vi "GeoData.vi"() -> ()   [LabVIEW 2017] (continued)
H1\n49649\t26055\tKingsley\tMI\tGrand Traverse County\tH1\n49684\t26055\tTraverse city\tMI\tGrand Traverse County\tH1\n49696\t26055\tTraverse city\tMI\tGrand Traverse County\tH1\n49666\t26055\tMayfield\tMI\tGrand Traverse County\tH1\n49683\t26055\tThompsonville\tMI\tGrand Traverse County\tH1\n48811\t26057\tCarson city\tMI\tGratiot County\tH1\n48862\t26057\tNorth star\tMI\tGratiot County\tH1\n48818\t26057\tCrystal\tMI\tGratiot County\tH1\n48830\t26057\tElm hall\tMI\tGratiot County\tH1\n48806\t26057\tAshley\tMI\tGratiot County\tH1\n48877\t26057\tRiverdale\tMI\tGratiot County\tH1\n48847\t26057\tIthaca\tMI\tGratiot County\tH1\n48874\t26057\tPompeii\tMI\tGratiot County\tH1\n48883\t26057\tShepherd\tMI\tGratiot County\tH1\n48891\t26057\tVestaburg\tMI\tGratiot County\tH1\n48879\t26057\tSaint johns\tMI\tGratiot County\tH1\n48889\t26057\tSumner\tMI\tGratiot County\tH1\n48637\t26057\tMerrill\tMI\tGratiot County\tH1\n48845\t26057\tHubbardston\tMI\tGratiot County\tH1\n48880\t26057\tSaint louis\tMI\tGratiot County\tH1\n48835\t26057\tFowler\tMI\tGratiot County\tH1\n48615\t26057\tBreckenridge\tMI\tGratiot County\tH1\n48832\t26057\tElwell\tMI\tGratiot County\tH1\n48801\t26057\tAlma\tMI\tGratiot County\tH1\n48662\t26057\tWheeler\tMI\tGratiot County\tH1\n48856\t26057\tMiddleton\tMI\tGratiot County\tH1\n48871\t26057\tPerrinton\tMI\tGratiot County\tH1\n48807\t26057\tBannister\tMI\tGratiot County\tH1\n48614\t26057\tBrant\tMI\tGratiot County\tH1\n48831\t26057\tElsie\tMI\tGratiot County\tH1\n49262\t26059\tNorth adams\tMI\tHillsdale County\tH1\n49255\t26059\tMontgomery\tMI\tHillsdale County\tH1\n49082\t26059\tQuincy\tMI\tHillsdale County\tH1\n49246\t26059\tHorton\tMI\tHillsdale County\tH1\n49220\t26059\tAddison\tMI\tHillsdale County\tH1\n49250\t26059\tJonesville\tMI\tHillsdale County\tH1\n49274\t26059\tReading\tMI\tHillsdale County\tH1\n49245\t26059\tHomer\tMI\tHillsdale County\tH1\n49282\t26059\tSomerset center\tMI\tHillsdale County\tH1\n49252\t26059\tLitchfield\tMI\tHillsdale County\tH1\n49233\t26059\tCement city\tMI\tHillsdale County\tH1\n49258\t26059\tMosherville\tMI\tHillsdale County\tH1\n49242\t26059\tHillsdale\tMI\tHillsdale County\tH1\n49266\t26059\tOsseo\tMI\tHillsdale County\tH1\n49249\t26059\tJerome\tMI\tHillsdale County\tH1\n49271\t26059\tPittsford\tMI\tHillsdale County\tH1\n49288\t26059\tWaldron\tMI\tHillsdale County\tH1\n49239\t26059\tFrontier\tMI\tHillsdale County\tH1\n49232\t26059\tCamden\tMI\tHillsdale County\tH1\n49227\t26059\tAllen\tMI\tHillsdale County\tH1\n49241\t26059\tHanover\tMI\tHillsdale County\tH1\n49247\t26059\tHudson\tMI\tHillsdale County\tH1\n49257\t26059\tMoscow\tMI\tHillsdale County\tH1\n49281\t26059\tSomerset\tMI\tHillsdale County\tH1\n49931\t26061\tHoughton\tMI\tHoughton County\tH1\n49901\t26061\tAhmeek\tMI\tHoughton County\tH1\n49916\t26061\tChassell\tMI\tHoughton County\tH1\n49967\t26061\tTrout creek\tMI\tHoughton County\tH1\n49921\t26061\tDodgeville\tMI\tHoughton County\tH1\n49930\t26061\tHancock\tMI\tHoughton County\tH1\n49905\t26061\tAtlantic mine\tMI\tHoughton County\tH1\n49963\t26061\tSouth range\tMI\tHoughton County\tH1\n49952\t26061\tNisula\tMI\tHoughton County\tH1\n49961\t26061\tSidnaw\tMI\tHoughton County\tH1\n49958\t26061\tPelkie\tMI\tHoughton County\tH1\n49917\t26061\tCopper city\tMI\tHoughton County\tH1\n49934\t26061\tHubbell\tMI\tHoughton County\tH1\n49945\t26061\tLake linden\tMI\tHoughton County\tH1\n49913\t26061\tCalumet\tMI\tHoughton County\tH1\n49805\t26061\tAllouez\tMI\tHoughton County\tH1\n49922\t26061\tDollar bay\tMI\tHoughton County\tH1\n49965\t26061\tToivola\tMI\tHoughton County\tH1\n49955\t26061\tPainesdale\tMI\tHoughton County\tH1\n48413\t26063\tBad axe\tMI\tHuron County\tH1\n48456\t26063\tMinden city\tMI\tHuron County\tH1\n48726\t26063\tCass city\tMI\tHuron County\tH1\n48720\t26063\tBay port\tMI\tHuron County\tH1\n48755\t26063\tPigeon\tMI\tHuron County\tH1\n48725\t26063\tCaseville\tMI\tHuron County\tH1\n48731\t26063\tElkton\tMI\tHuron County\tH1\n48735\t26063\tGagetown\tMI\tHuron County\tH1\n48467\t26063\tPort austin\tMI\tHuron County\tH1\n48470\t26063\tRuth\tMI\tHuron County\tH1\n48445\t26063\tKinde\tMI\tHuron County\tH1\n48759\t26063\tSebewaing\tMI\tHuron County\tH1\n48754\t26063\tOwendale\tMI\tHuron County\tH1\n48468\t26063\tPort hope\tMI\tHuron County\tH1\n48441\t26063\tHarbor beach\tMI\tHuron County\tH1\n48475\t26063\tUbly\tMI\tHuron County\tH1\n48432\t26063\tFilion\tMI\tHuron County\tH1\n48767\t26063\tUnionville\tMI\tHuron County\tH1\n49285\t26065\tStockbridge\tMI\tIngham County\tH1\n48826\t26065\tEast lansing\tMI\tIngham County\tH1\n48933\t26065\tLansing\tMI\tIngham County\tH1\n48805\t26065\tOkemos\tMI\tIngham County\tH1\n48864\t26065\tOkemos\tMI\tIngham County\tH1\n48840\t26065\tHaslett\tMI\tIngham County\tH1\n48824\t26065\tEast lansing\tMI\tIngham County\tH1\n48854\t26065\tMason\tMI\tIngham County\tH1\n48821\t26065\tDimondale\tMI\tIngham County\tH1\n48924\t26065\tLansing\tMI\tIngham County\tH1\n48911\t26065\tLansing\tMI\tIngham County\tH1\n48917\t26065\tLansing\tMI\tIngham County\tH1\n48825\t26065\tEast lansing\tMI\tIngham County\tH1\n48892\t26065\tWebberville\tMI\tIngham County\tH1\n48842\t26065\tHolt\tMI\tIngham County\tH1\n48819\t26065\tDansville\tMI\tIngham County\tH1\n48906\t26065\tLansing\tMI\tIngham County\tH1\n48909\t26065\tLansing\tMI\tIngham County\tH1\n48915\t26065\tLansing\tMI\tIngham County\tH1\n49264\t26065\tOnondaga\tMI\tIngham County\tH1\n48823\t26065\tEast lansing\tMI\tIngham County\tH1\n48910\t26065\tLansing\tMI\tIngham County\tH1\n48872\t26065\tPerry\tMI\tIngham County\tH1\n48901\t26065\tLansing\tMI\tIngham County\tH1\n48956\t26065\tLansing\tMI\tIngham County\tH1\n49251\t26065\tLeslie\tMI\tIngham County\tH1\n48827\t26065\tEaton rapids\tMI\tIngham County\tH1\n48912\t26065\tLansing\tMI\tIngham County\tH1\n48895\t26065\tWilliamston\tMI\tIngham County\tH1\n48849\t26067\tLake odessa\tMI\tIonia County\tH1\n48860\t26067\tMuir\tMI\tIonia County\tH1\n49331\t26067\tLowell\tMI\tIonia County\tH1\n49325\t26067\tFreeport\tMI\tIonia County\tH1\n48846\t26067\tIonia\tMI\tIonia County\tH1\n48875\t26067\tPortland\tMI\tIonia County\tH1\n48881\t26067\tSaranac\tMI\tIonia County\tH1\n48809\t26067\tBelding\tMI\tIonia County\tH1\n48838\t26067\tGreenville\tMI\tIonia County\tH1\n48890\t26067\tSunfield\tMI\tIonia County\tH1\n48834\t26067\tFenwick\tMI\tIonia County\tH1\n48815\t26067\tClarksville\tMI\tIonia County\tH1\n48865\t26067\tOrleans\tMI\tIonia County\tH1\n48873\t26067\tPewamo\tMI\tIonia County\tH1\n48870\t26067\tPalo\tMI\tIonia County\tH1\n48845\t26067\tHubbardston\tMI\tIonia County\tH1\n48894\t26067\tWestphalia\tMI\tIonia County\tH1\n48837\t26067\tGrand ledge\tMI\tIonia County\tH1\n48851\t26067\tLyons\tMI\tIonia County\tH1\n48861\t26067\tMulliken\tMI\tIonia County\tH1\n49302\t26067\tAlto\tMI\tIonia County\tH1\n48750\t26069\tOscoda\tMI\tIosco County\tH1\n48748\t26069\tNational city\tMI\tIosco County\tH1\n48770\t26069\tWhittemore\tMI\tIosco County\tH1\n48739\t26069\tHale\tMI\tIosco County\tH1\n48766\t26069\tTwining\tMI\tIosco County\tH1\n48761\t26069\tSouth branch\tMI\tIosco County\tH1\n48745\t26069\tMikado\tMI\tIosco County\tH1\n48738\t26069\tGreenbush\tMI\tIosco County\tH1\n48737\t26069\tGlennie\tMI\tIosco County\tH1\n48765\t26069\tTurner\tMI\tIosco County\tH1\n48730\t26069\tEast tawas\tMI\tIosco County\tH1\n48763\t26069\tTawas city\tMI\tIosco County\tH1\n48743\t26069\tLong lake\tMI\tIosco County\tH1\n49967\t26071\tTrout creek\tMI\tIron County\tH1\n49915\t26071\tCaspian\tMI\tIron County\tH1\n49927\t26071\tGaastra\tMI\tIron County\tH1\n49902\t26071\tAlpha\tMI\tIron County\tH1\n49920\t26071\tCrystal falls\tMI\tIron County\tH1\n49903\t26071\tAmasa\tMI\tIron County\tH1\n49879\t26071\tRepublic\tMI\tIron County\tH1\n49935\t26071\tIron river\tMI\tIron County\tH1\n49964\t26071\tStambaugh\tMI\tIron County\tH1\n48632\t26073\tLake\tMI\tIsabella County\tH1\n48804\t26073\tMount pleasant\tMI\tIsabella County\tH1\n49310\t26073\tBlanchard\tMI\tIsabella County\tH1\n49340\t26073\tRemus\tMI\tIsabella County\tH1\n49305\t26073\tBarryton\tMI\tIsabella County\tH1\n48618\t26073\tColeman\tMI\tIsabella County\tH1\n48877\t26073\tRiverdale\tMI\tIsabella County\tH1\n48893\t26073\tWeidman\tMI\tIsabella County\tH1\n48878\t26073\tRosebush\tMI\tIsabella County\tH1\n48622\t26073\tFarwell\tMI\tIsabella County\tH1\n48883\t26073\tShepherd\tMI\tIsabella County\tH1\n48891\t26073\tVestaburg\tMI\tIsabella County\tH1\n48858\t26073\tMount pleasant\tMI\tIsabella County\tH1\n48880\t26073\tSaint louis\tMI\tIsabella County\tH1\n48896\t26073\tWinn\tMI\tIsabella County\tH1\n48617\t26073\tClare\tMI\tIsabella County\tH1\n48801\t26073\tAlma\tMI\tIsabella County\tH1\n48829\t26073\tEdmore\tMI\tIsabella County\tH1\n48859\t26073\tMount pleasant\tMI\tIsabella County\tH1\n49224\t26075\tAlbion\tMI\tJackson County\tH1\n49202\t26075\tJackson\tMI\tJackson County\tH1\n49285\t26075\tStockbridge\tMI\tJackson County\tH1\n49272\t26075\tPleasant lake\tMI\tJackson County\tH1\n49203\t26075\tJackson\tMI\tJackson County\tH1\n49246\t26075\tHorton\tMI\tJackson County\tH1\n49204\t26075\tJackson\tMI\tJackson County\tH1\n49250\t26075\tJonesville\tMI\tJackson County\tH1\n49245\t26075\tHomer\tMI\tJackson County\tH1\n49201\t26075\tJackson\tMI\tJackson County\tH1\n49269\t26075\tParma\tMI\tJackson County\tH1\n49277\t26075\tRives junction\tMI\tJackson County\tH1\n49252\t26075\tLitchfield\tMI\tJackson County\tH1\n49284\t26075\tSpringport\tMI\tJackson County\tH1\n49259\t26075\tMunith\tMI\tJackson County\tH1\n49233\t26075\tCement city\tMI\tJackson County\tH1\n48158\t26075\tManchester\tMI\tJackson County\tH1\n49237\t26075\tConcord\tMI\tJackson County\tH1\n49254\t26075\tMichigan center\tMI\tJackson County\tH1\n49263\t26075\tNorvell\tMI\tJackson County\tH1\n48118\t26075\tChelsea\tMI\tJackson County\tH1\n49234\t26075\tClarklake\tMI\tJackson County\tH1\n49249\t26075\tJerome\tMI\tJackson County\tH1\n49261\t26075\tNapoleon\tMI\tJackson County\tH1\n49264\t26075\tOnondaga\tMI\tJackson County\tH1\n49241\t26075\tHanover\tMI\tJackson County\tH1\n49230\t26075\tBrooklyn\tMI\tJackson County\tH1\n49240\t26075\tGrass lake\tMI\tJackson County\tH1\n49251\t26075\tLeslie\tMI\tJackson County\tH1\n49283\t26075\tSpring arbor\tMI\tJackson County\tH1\n48827\t26075\tEaton rapids\tMI\tJackson County\tH1\n49004\t26077\tKalamazoo\tMI\tKalamazoo County\tH1\n49080\t26077\tPlainwell\tMI\tKalamazoo County\tH1\n49074\t26077\tNazareth\tMI\tKalamazoo County\tH1\n49009\t26077\tKalamazoo\tMI\tKalamazoo County\tH1\n49007\t26077\tKalamazoo\tMI\tKalamazoo County\tH1\n49083\t26077\tRichland\tMI\tKalamazoo County\tH1\n49087\t26077\tSchoolcraft\tMI\tKalamazoo County\tH1\n49003\t26077\tKalamazoo\tMI\tKalamazoo County\tH1\n49060\t26077\tHickory corners\tMI\tKalamazoo County\tH1\n49011\t26077\tAthens\tMI\tKalamazoo County\tH1\n49008\t26077\tKalamazoo\tMI\tKalamazoo County\tH1\n49072\t26077\tMendon\tMI\tKalamazoo County\tH1\n49005\t26077\tKalamazoo\tMI\tKalamazoo County\tH1\n49034\t26077\tClimax\tMI\tKalamazoo County\tH1\n49006\t26077\tKalamazoo\tMI\tKalamazoo County\tH1\n49015\t26077\tBattle creek\tMI\tKalamazoo County\tH1\n49001\t26077\tKalamazoo\tMI\tKalamazoo County\tH1\n49097\t26077\tVicksburg\tMI\tKalamazoo County\tH1\n49065\t26077\tLawton\tMI\tKalamazoo County\tH1\n49078\t26077\tOtsego\tMI\tKalamazoo County\tH1\n49052\t26077\tFulton\tMI\tKalamazoo County\tH1\n49053\t26077\tGalesburg\tMI\tKalamazoo County\tH1\n49081\t26077\tPortage\tMI\tKalamazoo County\tH1\n49041\t26077\tComstock\tMI\tKalamazoo County\tH1\n49017\t26077\tBattle creek\tMI\tKalamazoo County\tH1\n49037\t26077\tBattle creek\tMI\tKalamazoo County\tH1\n49012\t26077\tAugusta\tMI\tKalamazoo County\tH1\n49019\t26077\tKalamazoo\tMI\tKalamazoo County\tH1\n49024\t26077\tPortage\tMI\tKalamazoo County\tH1\n49002\t26077\tPortage\tMI\tKalamazoo County\tH1\n49048\t26077\tKalamazoo\tMI\tKalamazoo County\tH1\n49071\t26077\tMattawan\tMI\tKalamazoo County\tH1\n49088\t26077\tScotts\tMI\tKalamazoo County\tH1\n49077\t26077\tOshtemo\tMI\tKalamazoo County\tH1\n49690\t26079\tWilliamsburg\tMI\tKalkaska County\tH1\n49680\t26079\tSouth boardman\tMI\tKalkaska County\tH1\n49612\t26079\tAlden\tMI\tKalkaska County\tH1\n49633\t26079\tFife lake\tMI\tKalkaska County\tH1\n49659\t26079\tMancelona\tMI\tKalkaska County\tH1\n49738\t26079\tGrayling\tMI\tKalkaska County\tH1\n49646\t26079\tKalkaska\tMI\tKalkaska County\tH1\n49676\t26079\tRapid city\tMI\tKalkaska County\tH1\n49323\t26081\tDorr\tMI\tKent County\tH1\n49331\t26081\tLowell\tMI\tKent County\tH1\n49325\t26081\tFreeport\tMI\tKent County\tH1\n49418\t26081\tGrandville\tMI\tKent County\tH1\n49515\t26081\tGrand rapids\tMI\tKent County\tH1\n49514\t26081\tGrand rapids\tMI\tKent County\tH1\n49351\t26081\tRockford\tMI\tKent County\tH1\n49519\t26081\tWyoming\tMI\tKent County\tH1\n49507\t26081\tGrand rapids\tMI\tKent County\tH1\n49348\t26081\tWayland\tMI\tKent County\tH1\n49504\t26081\tGrand rapids\tMI\tKent County\tH1\n49518\t26081\tGrand rapids\tMI\tKent County\tH1\n49588\t26081\tGrand rapids\tMI\tKent County\tH1\n49315\t26081\tByron center\tMI\tKent County\tH1\n49330\t26081\tKent city\tMI\tKent County\tH1\n49316\t26081\tCaledonia\tMI\tKent County\tH1\n49534\t26081\tGrand rapids\tMI\tKent County\tH1\n49509\t26081\tWyoming\tMI\tKent County\tH1\n49508\t26081\tGrand rapids\tMI\tKent County\tH1\n49546\t26081\tGrand rapids\tMI\tKent County\tH1\n49544\t26081\tGrand rapids\tMI\tKent County\tH1\n49326\t26081\tGowen\tMI\tKent County\tH1\n48809\t26081\tBelding\tMI\tKent County\tH1\n48838\t26081\tGreenville\tMI\tKent County\tH1\n49319\t26081\tCedar springs\tMI\tKent County\tH1\n49506\t26081\tGrand rapids\tMI\tKent County\tH1\n49525\t26081\tGrand rapids\tMI\tKent County\tH1\n49345\t26081\tSparta\tMI\tKent County\tH1\n48815\t26081\tClarksville\tMI\tKent County\tH1\n49347\t26081\tTrufant\tMI\tKent County\tH1\n49321\t26081\tComstock park\tMI\tKent County\tH1\n49327\t26081\tGrant\tMI\tKent County\tH1\n49301\t26081\tAda\tMI\tKent County\tH1\n49512\t26081\tGrand rapids\tMI\tKent County\tH1\n49516\t26081\tGrand rapids\tMI\tKent County\tH1\n49343\t26081\tSand lake\tMI\tKent County\tH1\n49503\t26081\tGrand rapids\tMI\tKent County\tH1\n49435\t26081\tMarne\tMI\tKent County\tH1\n49510\t26081\tGrand rapids\tMI\tKent County\tH1\n49548\t26081\tGrand rapids\tMI\tKent County\tH1\n49341\t26081\tRockford\tMI\tKent County\tH1\n49333\t26081\tMiddleville\tMI\tKent County\tH1\n49403\t26081\tConklin\tMI\tKent County\tH1\n49501\t26081\tGrand rapids\tMI\tKent County\tH1\n49468\t26081\tGrandville\tMI\tKent County\tH1\n49560\t26081\tGrand rapids\tMI\tKent County\tH1\n49306\t26081\tBelmont\tMI\tKent County\tH1\n49302\t26081\tAlto\tMI\tKent County\tH1\n49318\t26081\tCasnovia\tMI\tKent County\tH1\n49505\t26081\tGrand rapids\tMI\tKent County\tH1\n49303\t26081\tBailey\tMI\tKent County\tH1\n49317\t26081\tCannonsburg\tMI\tKent County\tH1\n49901\t26083\tAhmeek\tMI\tKeweenaw County\tH1\n49950\t26083\tMohawk\tMI\tKeweenaw County\tH1\n49917\t26083\tCopper city\tMI\tKeweenaw County\tH1\n49918\t26083\tCopper harbor\tMI\tKeweenaw County\tH1\n49945\t26083\tLake linden\tMI\tKeweenaw County\tH1\n49913\t26083\tCalumet\tMI\tKeweenaw County\tH1\n49805\t26083\tAllouez\tMI\tKeweenaw County\tH1\n49677\t26085\tReed city\tMI\tLake County\tH1\n49304\t26085\tBaldwin\tMI\tLake County\tH1\n49644\t26085\tIrons\tMI\tLake County\tH1\n49623\t26085\tChase\tMI\tLake County\tH1\n49688\t26085\tTustin\tMI\tLake County\tH1\n49601\t26085\tCadillac\tMI\tLake County\tH1\n49642\t26085\tIdlewild\tMI\tLake County\tH1\n49656\t26085\tLuther\tMI\tLake County\tH1\n49655\t26085\tLeroy\tMI\tLake County\tH1\n49309\t26085\tBitely\tMI\tLake County\tH1\n49402\t26085\tBranch\tMI\tLake County\tH1\n48014\t26087\tCapac\tMI\tLapeer County\tH1\n48462\t26087\tOrtonville\tMI\tLapeer County\tH1\n48421\t26087\tColumbiaville\tMI\tLapeer County\tH1\n48440\t26087\tHadley\tMI\tLapeer County\tH1\n48444\t26087\tImlay city\tMI\tLapeer County\tH1\n48461\t26087\tNorth branch\tMI\tLapeer County\tH1\n48727\t26087\tClifford\tMI\tLapeer County\tH1\n48003\t26087\tAlmont\tMI\tLapeer County\tH1\n48760\t26087\tSilverwood\tMI\tLapeer County\tH1\n48412\t26087\tAttica\tMI\tLapeer County\tH1\n48455\t26087\tMetamora\tMI\tLapeer County\tH1\n48438\t26087\tGoodrich\tMI\tLapeer County\tH1\n48416\t26087\tBrown city\tMI\tLapeer County\tH1\n48453\t26087\tMarlette\tMI\tLapeer County\tH1\n48435\t26087\tFostoria\tMI\tLapeer County\tH1\n48744\t26087\tMayville\tMI\tLapeer County\tH1\n48464\t26087\tOtter lake\tMI\tLapeer County\tH1\n48463\t26087\tOtisville\tMI\tLapeer County\tH1\n48371\t26087\tOxford\tMI\tLapeer County\tH1\n48446\t26087\tLapeer\tMI\tLapeer County\tH1\n48423\t26087\tDavison\tMI\tLapeer County\tH1\n48428\t26087\tDryden\tMI\tLapeer County\tH1\n49650\t26089\tLake ann\tMI\tLeelanau County\tH1\n49621\t26089\tCedar\tMI\tLeelanau County\tH1\n49674\t26089\tOmena\tMI\tLeelanau County\tH1\n49664\t26089\tMaple city\tMI\tLeelanau County\tH1\n49653\t26089\tLake leelanau\tMI\tLeelanau County\tH1\n49654\t26089\tLeland\tMI\tLeelanau County\tH1\n49640\t26089\tHonor\tMI\tLeelanau County\tH1\n49682\t26089\tSuttons bay\tMI\tLeelanau County\tH1\n49684\t26089\tTraverse city\tMI\tLeelanau County\tH1\n49636\t26089\tGlen arbor\tMI\tLeelanau County\tH1\n49670\t26089\tNorthport\tMI\tLeelanau County\tH1\n49630\t26089\tEmpire\tMI\tLeelanau County\tH1\n49267\t26091\tOttawa lake\tMI\tLenawee County\tH1\n49228\t26091\tBlissfield\tMI\tLenawee County\tH1\n49253\t26091\tManitou beach\tMI\tLenawee County\tH1\n49220\t26091\tAddison\tMI\tLenawee County\tH1\n49235\t26091\tClayton\tMI\tLenawee County\tH1\n49268\t26091\tPalmyra\tMI\tLenawee County\tH1\n49229\t26091\tBritton\tMI\tLenawee County\tH1\n49287\t26091\tTipton\tMI\tLenawee County\tH1\n49233\t26091\tCement city\tMI\tLenawee County\tH1\n49256\t26091\tMorenci\tMI\tLenawee County\tH1\n49279\t26091\tSand creek\tMI\tLenawee County\tH1\n49238\t26091\tDeerfield\tMI\tLenawee County\tH1\n48160\t26091\tMilan\tMI\tLenawee County\tH1\n49248\t26091\tJasper\tMI\tLenawee County\tH1\n49288\t26091\tWaldron\tMI\tLenawee County\tH1\n49276\t26091\tRiga\tMI\tLenawee County\tH1\n48176\t26091\tSaline\tMI\tLenawee County\tH1\n49236\t26091\tClinton\tMI\tLenawee County\tH1\n49221\t26091\tAdrian\tMI\tLenawee County\tH1\n49230\t26091\tBrooklyn\tMI\tLenawee County\tH1\n49265\t26091\tOnsted\tMI\tLenawee County\tH1\n49247\t26091\tHudson\tMI\tLenawee County\tH1\n49286\t26091\tTecumseh\tMI\tLenawee County\tH1\n49289\t26091\tWeston\tMI\tLenawee County\tH1\n48137\t26093\tGregory\tMI\tLivingston County\tH1\n48178\t26093\tSouth lyon\tMI\tLivingston County\tH1\n48442\t26093\tHolly\tMI\tLivingston County\tH1\n49285\t26093\tStockbridge\tMI\tLivingston County\tH1\n48353\t26093\tHartland\tMI\tLivingston County\tH1\n48451\t26093\tLinden\tMI\tLivingston County\tH1\n48844\t26093\tHowell\tMI\tLivingston County\tH1\n48816\t26093\tCohoctah\tMI\tLivingston County\tH1\n48169\t26093\tPinckney\tMI\tLivingston County\tH1\n48189\t26093\tWhitmore lake\tMI\tLivingston County\tH1\n48430\t26093\tFenton\tMI\tLivingston County\tH1\n48114\t26093\tBrighton\tMI\tLivingston County\tH1\n48418\t26093\tByron\tMI\tLivingston County\tH1\n48892\t26093\tWebberville\tMI\tLivingston County\tH1\n48116\t26093\tBrighton\tMI\tLivingston County\tH1\n48380\t26093\tMilford\tMI\tLivingston County\tH1\n48836\t26093\tFowlerville\tMI\tLivingston County\tH1\n48872\t26093\tPerry\tMI\tLivingston County\tH1\n48855\t26093\tHowell\tMI\tLivingston County\tH1\n48843\t26093\tHowell\tMI\tLivingston County\tH1\n48139\t26093\tHamburg\tMI\tLivingston County\tH1\n48143\t26093\tLakeland\tMI\tLivingston County\tH1\n49853\t26095\tMc millan\tMI\tLuce County\tH1\n49868\t26095\tNewberry\tMI\tLuce County\tH1\n49762\t26097\tNaubinway\tMI\tMackinac County\tH1\n49781\t26097\tSaint ignace\tMI\tMackinac County\tH1\n49853\t26097\tMc millan\tMI\tMackinac County\tH1\n49780\t26097\tRudyard\tMI\tMackinac County\tH1\n49757\t26097\tMackinac island\tMI\tMackinac County\tH1\n49760\t26097\tMoran\tMI\tMackinac County\tH1\n49719\t26097\tCedarville\tMI\tMackinac County\tH1\n49745\t26097\tHessel\tMI\tMackinac County\tH1\n49820\t26097\tCurtis\tMI\tMackinac County\tH1\n49827\t26097\tEngadine\tMI\tMackinac County\tH1\n49836\t26097\tGermfask\tMI\tMackinac County\tH1\n49775\t26097\tPointe aux pins\tMI\tMackinac County\tH1\n49838\t26097\tGould city\tMI\tMackinac County\tH1\n49774\t26097\tPickford\tMI\tMackinac County\tH1\n48021\t26099\tEastpointe\tMI\tMacomb County\tH1\n48044\t26099\tMacomb\tMI\tMacomb County\tH1\n48041\t26099\tMemphis\tMI\tMacomb County\tH1\n48065\t26099\tRomeo\tMI\tMacomb County\tH1\n48080\t26099\tSaint clair shores\tMI\tMacomb County\tH1\n48094\t26099\tWashington\tMI\tMacomb County\tH1\n48085\t26099\tTroy\tMI\tMacomb County\tH1\n48318\t26099\tUtica\tMI\tMacomb County\tH1\n48038\t26099\tClinton township\tMI\tMacomb County\tH1\n48089\t26099\tWarren\tMI\tMacomb County\tH1\n48236\t26099\tGrosse pointe\tMI\tMacomb County\tH1\n48066\t26099\tRoseville\tMI\tMacomb County\tH1\n48050\t26099\tNew haven\tMI\tMacomb County\tH1\n48048\t26099\tNew haven\tMI\tMacomb County\tH1\n48042\t26099\tMacomb\tMI\tMacomb County\tH1\n48312\t26099\tSterling heights\tMI\tMacomb County\tH1\n48081\t26099\tSaint clair shores\tMI\tMacomb County\tH1\n48051\t26099\tNew baltimore\tMI\tMacomb County\tH1\n48047\t26099\tNew baltimore\tMI\tMacomb County\tH1\n48088\t26099\tWarren\tMI\tMacomb County\tH1\n48015\t26099\tCenter line\tMI\tMacomb County\tH1\n48036\t26099\tClinton township\tMI\tMacomb County\tH1\n48313\t26099\tSterling heights\tMI\tMacomb County\tH1\n48062\t26099\tRichmond\tMI\tMacomb County\tH1\n48092\t26099\tWarren\tMI\tMacomb County\tH1\n48096\t26099\tRay\tMI\tMacomb County\tH1\n48026\t26099\tFraser\tMI\tMacomb County\tH1\n48310\t26099\tSterling heights\tMI\tMacomb County\tH1\n48306\t26099\tRochester\tMI\tMacomb County\tH1\n48316\t26099\tUtica\tMI\tMacomb County\tH1\n48095\t26099\tWashington\tMI\tMacomb County\tH1\n48317\t26099\tUtica\tMI\tMacomb County\tH1\n48035\t26099\tClinton township\tMI\tMacomb County\tH1\n48315\t26099\tUtica\tMI\tMacomb County\tH1\n48082\t26099\tSaint clair shores\tMI\tMacomb County\tH1\n48091\t26099\tWarren\tMI\tMacomb County\tH1\n48093\t26099\tWarren\tMI\tMacomb County\tH1\n48046\t26099\tMount clemens\tMI\tMacomb County\tH1\n48005\t26099\tArmada\tMI\tMacomb County\tH1\n48043\t26099\tMount clemens\tMI\tMacomb County\tH1\n48314\t26099\tSterling heights\tMI\tMacomb County\tH1\n48311\t26099\tSterling heights\tMI\tMacomb County\tH1\n48045\t26099\tHarrison township\tMI\tMacomb County\tH1\n48090\t26099\tWarren\tMI\tMacomb County\tH1\n49638\t26101\tHarrietta\tMI\tManistee County\tH1\n49619\t26101\tBrethren\tMI\tManistee County\tH1\n49634\t26101\tFiler city\tMI\tManistee County\tH1\n49644\t26101\tIrons\tMI\tManistee County\tH1\n49411\t26101\tFree soil\tMI\tManistee County\tH1\n49660\t26101\tManistee\tMI\tManistee County\tH1\n49689\t26101\tWellston\tMI\tManistee County\tH1\n49626\t26101\tEastlake\tMI\tManistee County\tH1\n49675\t26101\tOnekama\tMI\tManistee County\tH1\n49668\t26101\tMesick\tMI\tManistee County\tH1\n49625\t26101\tCopemish\tMI\tManistee County\tH1\n49614\t26101\tBear lake\tMI\tManistee County\tH1\n49616\t26101\tBenzonia\tMI\tManistee County\tH1\n49613\t26101\tArcadia\tMI\tManistee County\tH1\n49645\t26101\tKaleva\tMI\tManistee County\tH1\n49683\t26101\tThompsonville\tMI\tManistee County\tH1\n49814\t26103\tChampion\tMI\tMarquette County\tH1\n49878\t26103\tRapid river\tMI\tMarquette County\tH1\n49865\t26103\tNational mine\tMI\tMarquette County\tH1\n49880\t26103\tRock\tMI\tMarquette County\tH1\n49855\t26103\tMarquette\tMI\tMarquette County\tH1\n49833\t26103\tLittle lake\tMI\tMarquette County\tH1\n49885\t26103\tSkandia\tMI\tMarquette County\tH1\n49819\t26103\tArnold\tMI\tMarquette County\tH1\n49808\t26103\tBig bay\tMI\tMarquette County\tH1\n49871\t26103\tPalmer\tMI\tMarquette County\tH1\n49841\t26103\tGwinn\tMI\tMarquette County\tH1\n49849\t26103\tIshpeming\tMI\tMarquette County\tH1\n49879\t26103\tRepublic\tMI\tMarquette County\tH1\n49861\t26103\tMichigamme\tMI\tMarquette County\tH1\n49818\t26103\tCornell\tMI\tMarquette County\tH1\n49822\t26103\tDeerton\tMI\tMarquette County\tH1\n49866\t26103\tNegaunee\tMI\tMarquette County\tH1\n49449\t26105\tPentwater\tMI\tMason County\tH1\n49410\t26105\tFountain\tMI\tMason County\tH1\n49405\t26105\tCuster\tMI\tMason County\tH1\n49458\t26105\tWalhalla\tMI\tMason County\tH1\n49644\t26105\tIrons\tMI\tMason County\tH1\n49411\t26105\tFree soil\tMI\tMason County\tH1\n49660\t26105\tManistee\tMI\tMason County\tH1\n49420\t26105\tHart\tMI\tMason County\tH1\n49431\t26105\tLudington\tMI\tMason County\tH1\n49454\t26105\tScottville\tMI\tMason County\tH1\n49402\t26105\tBranch\tMI\tMason County\tH1\n49310\t26107\tBlanchard\tMI\tMecosta County\tH1\n49329\t26107\tHoward city\tMI\tMecosta County\tH1\n49340\t26107\tRemus\tMI\tMecosta County\tH1\n49342\t26107\tRodney\tMI\tMecosta County\tH1\n49305\t26107\tBarryton\tMI\tMecosta County\tH1\n49337\t26107\tNewaygo\tMI\tMecosta County\tH1\n49307\t26107\tBig rapids\tMI\tMecosta County\tH1\n48850\t26107\tLakeview\tMI\tMecosta County\tH1\n49679\t26107\tSears\tMI\tMecosta County\tH1\n49346\t26107\tStanwood\tMI\tMecosta County\tH1\n49332\t26107\tMecosta\tMI\tMecosta County\tH1\n49639\t26107\tHersey\tMI\tMecosta County\tH1\n49338\t26107\tParis\tMI\tMecosta County\tH1\n48886\t26107\tSix lakes\tMI\tMecosta County\tH1\n49336\t26107\tMorley\tMI\tMecosta County\tH1\n49320\t26107\tChippewa lake\tMI\tMecosta County\tH1\n49631\t26107\tEvart\tMI\tMecosta County\tH1\n49847\t26109\tHermansville\tMI\tMenominee County\tH1\n49887\t26109\tStephenson\tMI\tMenominee County\tH1\n49893\t26109\tWallace\tMI\tMenominee County\tH1\n49858\t26109\tMenominee\tMI\tMenominee County\tH1\n49821\t26109\tDaggett\tMI\tMenominee County\tH1\n49812\t26109\tCarney\tMI\tMenominee County\tH1\n49874\t26109\tPowers\tMI\tMenominee County\tH1\n49807\t26109\tBark river\tMI\tMenominee County\tH1\n49896\t26109\tWilson\tMI\tMenominee County\tH1\n49863\t26109\tNadeau\tMI\tMenominee County\tH1\n49845\t26109\tHarris\tMI\tMenominee County\tH1\n49873\t26109\tPerronville\tMI\tMenominee County\tH1\n49848\t26109\tIngalls\tMI\tMenominee County\tH1\n49886\t26109\tSpalding\tMI\tMenominee County\tH1\n49892\t26109\tVulcan\tMI\tMenominee County\tH1\n48642\t26111\tMidland\tMI\tMidland County\tH1\n48623\t26111\tFreeland\tMI\tMidland County\tH1\n48620\t26111\tEdenville\tMI\tMidland County\tH1\n48640\t26111\tMidland\tMI\tMidland County\tH1\n48628\t26111\tHope\tMI\tMidland County\tH1\n48612\t26111\tBeaverton\tMI\tMidland County\tH1\n48618\t26111\tColeman\tMI\tMidland County\tH1\n48634\t26111\tLinwood\tMI\tMidland County\tH1\n48674\t26111\tMidland\tMI\tMidland County\tH1\n48883\t26111\tShepherd\tMI\tMidland County\tH1\n48626\t26111\tHemlock\tMI\tMidland County\tH1\n48637\t26111\tMerrill\tMI\tMidland County\tH1\n48858\t26111\tMount pleasant\tMI\tMidland County\tH1\n48880\t26111\tSaint louis\tMI\tMidland County\tH1\n48641\t26111\tMidland\tMI\tMidland County\tH1\n48667\t26111\tMidland\tMI\tMidland County\tH1\n48652\t26111\tRhodes\tMI\tMidland County\tH1\n48615\t26111\tBreckenridge\tMI\tMidland County\tH1\n48657\t26111\tSanford\tMI\tMidland County\tH1\n48662\t26111\tWheeler\tMI\tMidland County\tH1\n48670\t26111\tMidland\tMI\tMidland County\tH1\n49651\t26113\tLake city\tMI\tMissaukee County\tH1\n49633\t26113\tFife lake\tMI\tMissaukee County\tH1\n49665\t26113\tMarion\tMI\tMissaukee County\tH1\n49667\t26113\tMerritt\tMI\tMissaukee County\tH1\n49601\t26113\tCadillac\tMI\tMissaukee County\tH1\n48625\t26113\tHarrison\tMI\tMissaukee County\tH1\n49663\t26113\tManton\tMI\tMissaukee County\tH1\n49632\t26113\tFalmouth\tMI\tMissaukee County\tH1\n49657\t26113\tMc bain\tMI\tMissaukee County\tH1\n49267\t26115\tOttawa lake\tMI\tMonroe County\tH1\n48111\t26115\tBelleville\tMI\tMonroe County\tH1\n48134\t26115\tFlat rock\tMI\tMonroe County\tH1\n48131\t26115\tDundee\tMI\tMonroe County\tH1\n49228\t26115\tBlissfield\tMI\tMonroe County\tH1\n48144\t26115\tLambertville\tMI\tMonroe County\tH1\n48164\t26115\tNew boston\tMI\tMonroe County\tH1\n48161\t26115\tMonroe\tMI\tMonroe County\tH1\n48166\t26115\tNewport\tMI\tMonroe County\tH1\n48117\t26115\tCarleton\tMI\tMonroe County\tH1\n49229\t26115\tBritton\tMI\tMonroe County\tH1\n49270\t26115\tPetersburg\tMI\tMonroe County\tH1\n48133\t26115\tErie\tMI\tMonroe County\tH1\n48145\t26115\tLa salle\tMI\tMonroe County\tH1\n48191\t26115\tWillis\tMI\tMonroe County\tH1\n49238\t26115\tDeerfield\tMI\tMonroe County\tH1\n48160\t26115\tMilan\tMI\tMonroe County\tH1\n49276\t26115\tRiga\tMI\tMonroe County\tH1\n48162\t26115\tMonroe\tMI\tMonroe County\tH1\n48159\t26115\tMaybee\tMI\tMonroe County\tH1\n48182\t26115\tTemperance\tMI\tMonroe County\tH1\n48177\t26115\tSamaria\tMI\tMonroe County\tH1\n48179\t26115\tSouth rockwood\tMI\tMonroe County\tH1\n48157\t26115\tLuna pier\tMI\tMonroe County\tH1\n48140\t26115\tIda\tMI\tMonroe County\tH1\n48888\t26117\tStanton\tMI\tMontcalm County\tH1\n49310\t26117\tBlanchard\tMI\tMontcalm County\tH1\n49329\t26117\tHoward city\tMI\tMontcalm County\tH1\n48811\t26117\tCarson city\tMI\tMontcalm County\tH1\n49322\t26117\tCoral\tMI\tMontcalm County\tH1\n49337\t26117\tNewaygo\tMI\tMontcalm County\tH1\n48818\t26117\tCrystal\tMI\tMontcalm County\tH1\n49326\t26117\tGowen\tMI\tMontcalm County\tH1\n48877\t26117\tRiverdale\tMI\tMontcalm County\tH1\n48812\t26117\tCedar lake\tMI\tMontcalm County\tH1\n48809\t26117\tBelding\tMI\tMontcalm County\tH1\n48850\t26117\tLakeview\tMI\tMontcalm County\tH1\n48838\t26117\tGreenville\tMI\tMontcalm County\tH1\n48834\t26117\tFenwick\tMI\tMontcalm County\tH1\n49347\t26117\tTrufant\tMI\tMontcalm County\tH1\n48891\t26117\tVestaburg\tMI\tMontcalm County\tH1\n48884\t26117\tSheridan\tMI\tMontcalm County\tH1\n49343\t26117\tSand lake\tMI\tMontcalm County\tH1\n49339\t26117\tPierson\tMI\tMontcalm County\tH1\n48889\t26117\tSumner\tMI\tMontcalm County\tH1\n48852\t26117\tMcbrides\tMI\tMontcalm County\tH1\n48845\t26117\tHubbardston\tMI\tMontcalm County\tH1\n48885\t26117\tSidney\tMI\tMontcalm County\tH1\n48829\t26117\tEdmore\tMI\tMontcalm County\tH1\n48886\t26117\tSix lakes\tMI\tMontcalm County\tH1\n49336\t26117\tMorley\tMI\tMontcalm County\tH1\n49709\t26119\tAtlanta\tMI\tMontmorency County\tH1\n49746\t26119\tHillman\tMI\tMontmorency County\tH1\n49756\t26119\tLewiston\tMI\tMontmorency County\tH1\n49751\t26119\tJohannesburg\tMI\tMontmorency County\tH1\n48619\t26119\tComins\tMI\tMontmorency County\tH1\n49437\t26121\tMontague\tMI\tMuskegon County\tH1\n49456\t26121\tSpring lake\tMI\tMuskegon County\tH1\n49440\t26121\tMuskegon\tMI\tMuskegon County\tH1\n49415\t26121\tFruitport\tMI\tMuskegon County\tH1\n49330\t26121\tKent city\tMI\tMuskegon County\tH1\n49425\t26121\tHolton\tMI\tMuskegon County\tH1\n49445\t26121\tMuskegon\tMI\tMuskegon County\tH1\n49444\t26121\tMuskegon\tMI\tMuskegon County\tH1\n49461\t26121\tWhitehall\tMI\tMuskegon County\tH1\n49448\t26121\tNunica\tMI\tMuskegon County\tH1\n49327\t26121\tGrant\tMI\tMuskegon County\tH1\n49441\t26121\tMuskegon\tMI\tMuskegon County\tH1\n49404\t26121\tCoopersville\tMI\tMuskegon County\tH1\n49403\t26121\tConklin\tMI\tMuskegon County\tH1\n49443\t26121\tMuskegon\tMI\tMuskegon County\tH1\n49318\t26121\tCasnovia\tMI\tMuskegon County\tH1\n49442\t26121\tMuskegon\tMI\tMuskegon County\tH1\n49412\t26121\tFremont\tMI\tMuskegon County\tH1\n49457\t26121\tTwin lake\tMI\tMuskegon County\tH1\n49451\t26121\tRavenna\tMI\tMuskegon County\tH1\n49303\t26121\tBailey\tMI\tMuskegon County\tH1\n49329\t26123\tHoward city\tMI\tNewaygo County\tH1\n49677\t26123\tReed city\tMI\tNewaygo County\tH1\n49337\t26123\tNewaygo\tMI\tNewaygo County\tH1\n49307\t26123\tBig rapids\tMI\tNewaygo County\tH1\n49330\t26123\tKent city\tMI\tNewaygo County\tH1\n49349\t26123\tWhite cloud\tMI\tNewaygo County\tH1\n49425\t26123\tHolton\tMI\tNewaygo County\tH1\n49421\t26123\tHesperia\tMI\tNewaygo County\tH1\n49312\t26123\tBrohman\tMI\tNewaygo County\tH1\n49327\t26123\tGrant\tMI\tNewaygo County\tH1\n49346\t26123\tStanwood\tMI\tNewaygo County\tH1\n49343\t26123\tSand lake\tMI\tNewaygo County\tH1\n49339\t26123\tPierson\tMI\tNewaygo County\tH1\n49413\t26123\tFremont\tMI\tNewaygo County\tH1\n49459\t26123\tWalkerville\tMI\tNewaygo County\tH1\n49309\t26123\tBitely\tMI\tNewaygo County\tH1\n49338\t26123\tParis\tMI\tNewaygo County\tH1\n49336\t26123\tMorley\tMI\tNewaygo County\tH1\n49412\t26123\tFremont\tMI\tNewaygo County\tH1\n49457\t26123\tTwin lake\tMI\tNewaygo County\tH1\n49451\t26123\tRavenna\tMI\tNewaygo County\tH1\n49303\t26123\tBailey\tMI\tNewaygo County\tH1\n48178\t26125\tSouth lyon\tMI\tOakland County\tH1\n48071\t26125\tMadison heights\tMI\tOakland County\tH1\n48072\t26125\tBerkley\tMI\tOakland County\tH1\n48085\t26125\tTroy\tMI\tOakland County\tH1\n48346\t26125\tClarkston\tMI\tOakland County\tH1\n48348\t26125\tClarkston\tMI\tOakland County\tH1\n48342\t26125\tPontiac\tMI\tOakland County\tH1\n48370\t26125\tOxford\tMI\tOakland County\tH1\n48462\t26125\tOrtonville\tMI\tOakland County\tH1\n48442\t26125\tHolly\tMI\tOakland County\tH1\n48068\t26125\tRoyal oak\tMI\tOakland County\tH1\n48009\t26125\tBirmingham\tMI\tOakland County\tH1\n48033\t26125\tSouthfield\tMI\tOakland County\tH1\n48099\t26125\tTroy\tMI\tOakland County\tH1\n48220\t26125\tFerndale\tMI\tOakland County\tH1\n48360\t26125\tLake orion\tMI\tOakland County\tH1\n48374\t26125\tNovi\tMI\tOakland County\tH1\n48383\t26125\tWhite lake\tMI\tOakland County\tH1\n48331\t26125\tFarmington\tMI\tOakland County\tH1\n48357\t26125\tHighland\tMI\tOakland County\tH1\n48363\t26125\tOakland\tMI\tOakland County\tH1\n48037\t26125\tSouthfield\tMI\tOakland County\tH1\n48165\t26125\tNew hudson\tMI\tOakland County\tH1\n48237\t26125\tOak park\tMI\tOakland County\tH1\n48302\t26125\tBloomfield hills\tMI\tOakland County\tH1\n48329\t26125\tWaterford\tMI\tOakland County\tH1\n48324\t26125\tWest bloomfield\tMI\tOakland County\tH1\n48320\t26125\tKeego harbor\tMI\tOakland County\tH1\n48430\t26125\tFenton\tMI\tOakland County\tH1\n48025\t26125\tFranklin\tMI\tOakland County\tH1\n48167\t26125\tNorthville\tMI\tOakland County\tH1\n48335\t26125\tFarmington\tMI\tOakland County\tH1\n48455\t26125\tMetamora\tMI\tOakland County\tH1\n48361\t26125\tLake orion\tMI\tOakland County\tH1\n48333\t26125\tFarmington\tMI\tOakland County\tH1\n48330\t26125\tDrayton plains\tMI\tOakland County\tH1\n48017\t26125\tClawson\tMI\tOakland County\tH1\n48301\t26125\tBloomfield hills\tMI\tOakland County\tH1\n48304\t26125\tBloomfield hills\tMI\tOakland County\tH1\n48307\t26125\tRochester\tMI\tOakland County\tH1\n48309\t26125\tRochester\tMI\tOakland County\tH1\n48067\t26125\tRoyal oak\tMI\tOakland County\tH1\n48069\t26125\tPleasant ridge\tMI\tOakland County\tH1\n48341\t26125\tPontiac\tMI\tOakland County\tH1\n48323\t26125\tWest bloomfield\tMI\tOakland County\tH1\n48381\t26125\tMilford\tMI\tOakland County\tH1\n48326\t26125\tAuburn hills\tMI\tOakland County\tH1\n48386\t26125\tWhite lake\tMI\tOakland County\tH1\n48359\t26125\tLake orion\tMI\tOakland County\tH1\n48377\t26125\tNovi\tMI\tOakland County\tH1\n48321\t26125\tAuburn hills\tMI\tOakland County\tH1\n48347\t26125\tClarkston\tMI\tOakland County\tH1\n48306\t26125\tRochester\tMI\tOakland County\tH1\n48073\t26125\tRoyal oak\tMI\tOakland County\tH1\n48076\t26125\tSouthfield\tMI\tOakland County\tH1\n48075\t26125\tSouthfield\tMI\tOakland County\tH1\n48362\t26125\tLake orion\tMI\tOakland County\tH1\n48322\t26125\tWest bloomfield\tMI\tOakland County\tH1\n48317\t26125\tUtica\tMI\tOakland County\tH1\n48356\t26125\tHighland\tMI\tOakland County\tH1\n48375\t26125\tNovi\tMI\tOakland County\tH1\n48390\t26125\tWalled lake\tMI\tOakland County\tH1\n48393\t26125\tWixom\tMI\tOakland County\tH1\n48382\t26125\tCommerce township\tMI\tOakland County\tH1\n48387\t26125\tUnion lake\tMI\tOakland County\tH1\n48028\t26125\tHarsens island\tMI\tOakland County\tH1\n48034\t26125\tSouthfield\tMI\tOakland County\tH1\n48098\t26125\tTroy\tMI\tOakland County\tH1\n48219\t26125\tDetroit\tMI\tOakland County\tH1\n48371\t26125\tOxford\tMI\tOakland County\tH1\n48336\t26125\tFarmington\tMI\tOakland County\tH1\n48340\t26125\tPontiac\tMI\tOakland County\tH1\n48367\t26125\tLeonard\tMI\tOakland County\tH1\n48350\t26125\tDavisburg\tMI\tOakland County\tH1\n48327\t26125\tWaterford\tMI\tOakland County\tH1\n48380\t26125\tMilford\tMI\tOakland County\tH1\n48439\t26125\tGrand blanc\tMI\tOakland County\tH1\n48070\t26125\tHuntington woods\tMI\tOakland County\tH1\n48325\t26125\tWest bloomfield\tMI\tOakland County\tH1\n48376\t26125\tNovi\tMI\tOakland County\tH1\n48332\t26125\tFarmington\tMI\tOakland County\tH1\n48012\t26125\tBirmingham\tMI\tOakland County\tH1\n48030\t26125\tHazel park\tMI\tOakland County\tH1\n48083\t26125\tTroy\tMI\tOakland County\tH1\n48084\t26125\tTroy\tMI\tOakland County\tH1\n48334\t26125\tFarmington\tMI\tOakland County\tH1\n48328\t26125\tWaterford\tMI\tOakland County\tH1\n48343\t26125\tPontiac\tMI\tOakland County\tH1\n48303\t26125\tBloomfield hills\tMI\tOakland County\tH1\n48308\t26125\tRochester\tMI\tOakland County\tH1\n48428\t26125\tDryden\tMI\tOakland County\tH1\n48366\t26125\tLakeville\tMI\tOakland County\tH1\n49437\t26127\tMontague\tMI\tOceana County\tH1\n49449\t26127\tPentwater\tMI\tOceana County\tH1\n49436\t26127\tMears\tMI\tOceana County\tH1\n49425\t26127\tHolton\tMI\tOceana County\tH1\n49446\t26127\tNew era\tMI\tOceana County\tH1\n49421\t26127\tHesperia\tMI\tOceana County\tH1\n49459\t26127\tWalkerville\tMI\tOceana County\tH1\n49452\t26127\tRothbury\tMI\tOceana County\tH1\n49420\t26127\tHart\tMI\tOceana County\tH1\n49412\t26127\tFremont\tMI\tOceana County\tH1\n49402\t26127\tBranch\tMI\tOceana County\tH1\n49455\t26127\tShelby\tMI\tOceana County\tH1\n48624\t26129\tGladwin\tMI\tOgemaw County\tH1\n48654\t26129\tRose city\tMI\tOgemaw County\tH1\n48770\t26129\tWhittemore\tMI\tOgemaw County\tH1\n48739\t26129\tHale\tMI\tOgemaw County\tH1\n48756\t26129\tPrescott\tMI\tOgemaw County\tH1\n48659\t26129\tSterling\tMI\tOgemaw County\tH1\n48761\t26129\tSouth branch\tMI\tOgemaw County\tH1\n48610\t26129\tAlger\tMI\tOgemaw County\tH1\n48635\t26129\tLupton\tMI\tOgemaw County\tH1\n48661\t26129\tWest branch\tMI\tOgemaw County\tH1\n49948\t26131\tMass city\tMI\tOntonagon County\tH1\n49967\t26131\tTrout creek\tMI\tOntonagon County\tH1\n49971\t26131\tWhite pine\tMI\tOntonagon County\tH1\n49947\t26131\tMarenisco\tMI\tOntonagon County\tH1\n49953\t26131\tOntonagon\tMI\tOntonagon County\tH1\n49960\t26131\tRockland\tMI\tOntonagon County\tH1\n49929\t26131\tGreenland\tMI\tOntonagon County\tH1\n49965\t26131\tToivola\tMI\tOntonagon County\tH1\n49912\t26131\tBruce crossing\tMI\tOntonagon County\tH1\n49925\t26131\tEwen\tMI\tOntonagon County\tH1\n49910\t26131\tBergland\tMI\tOntonagon County\tH1\n48632\t26133\tLake\tMI\tOsceola County\tH1\n49677\t26133\tReed city\tMI\tOsceola County\tH1\n49665\t26133\tMarion\tMI\tOsceola County\tH1\n49688\t26133\tTustin\tMI\tOsceola County\tH1\n49679\t26133\tSears\tMI\tOsceola County\tH1\n49655\t26133\tLeroy\tMI\tOsceola County\tH1\n49639\t26133\tHersey\tMI\tOsceola County\tH1\n49338\t26133\tParis\tMI\tOsceola County\tH1\n49657\t26133\tMc bain\tMI\tOsceola County\tH1\n49631\t26133\tEvart\tMI\tOsceola County\tH1\n48728\t26135\tCurran\tMI\tOscoda County\tH1\n48621\t26135\tFairview\tMI\tOscoda County\tH1\n48654\t26135\tRose city\tMI\tOscoda County\tH1\n48761\t26135\tSouth branch\tMI\tOscoda County\tH1\n48647\t26135\tMio\tMI\tOscoda County\tH1\n49756\t26135\tLewiston\tMI\tOscoda County\tH1\n48619\t26135\tComins\tMI\tOscoda County\tH1\n48636\t26135\tLuzerne\tMI\tOscoda County\tH1\n49797\t26137\tWaters\tMI\tOtsego County\tH1\n49795\t26137\tVanderbilt\tMI\tOtsego County\tH1\n49738\t26137\tGrayling\tMI\tOtsego County\tH1\n49735\t26137\tGaylord\tMI\tOtsego County\tH1\n49756\t26137\tLewiston\tMI\tOtsego County\tH1\n49730\t26137\tElmira\tMI\tOtsego County\tH1\n49733\t26137\tFrederic\tMI\tOtsego County\tH1\n49751\t26137\tJohannesburg\tMI\tOtsego County\tH1\n49734\t26137\tGaylord\tMI\tOtsego County\tH1\n49323\t26139\tDorr\tMI\tOttawa County\tH1\n49418\t26139\tGrandville\tMI\tOttawa County\tH1\n49423\t26139\tHolland\tMI\tOttawa County\tH1\n49426\t26139\tHudsonville\tMI\tOttawa County\tH1\n49456\t26139\tSpring lake\tMI\tOttawa County\tH1\n49409\t26139\tFerrysburg\t
